vi "Write Single Coil.vi"(8 "error in":errorcluster, 9 "coil value":bool, 10 "address":u16, 11 "device data model in":refnum<class "Standard Data Model.lvclass">) -> (0 "error out":errorcluster, 3 "device data model out":refnum<class "Standard Data Model.lvclass">)   [LabVIEW 2021, in "Standard Data Model.lvclass"]
doc: "Writes the value of a single coil."
uses:
  Standard Data Model.lvclass
  Standard Data Model.lvclass/Standard Data Model.ctl
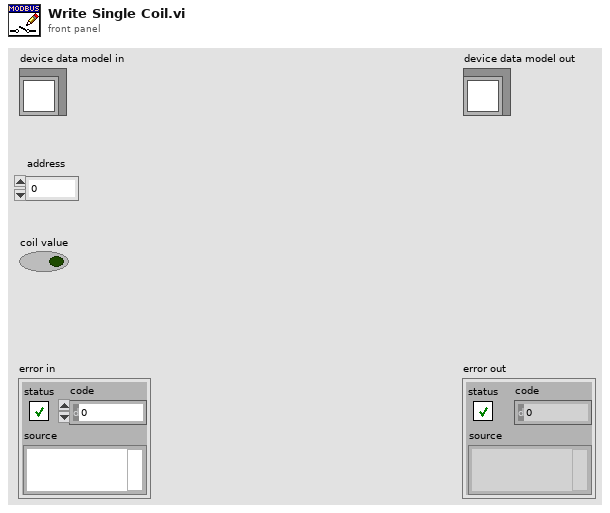
[diagram p1: front panel]
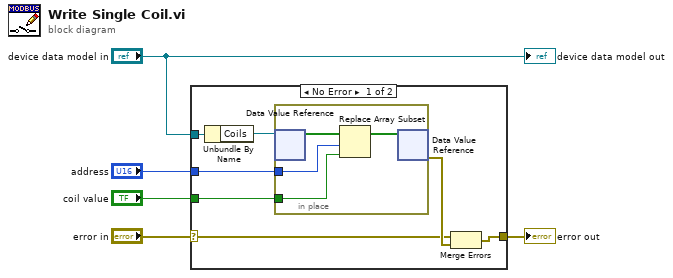
[diagram p0: block diagram]
diagram:
  n1 = case shown="No Error" "error in" {
    selector: "error in" -> [w6 w17]
    tunnel: "device data model in" -> [w12 _]
    tunnel: "coil value" -> [w10 _]
    tunnel: [w8 w17] -> w3
    tunnel: "address" -> [w7 _]
    frame No Error {
      n2 = Unbundle By Name(w12) -> ("Coils"=w11:refnum<data-value>)
      n3 = in-place {
        in-place-border: w10 -> [w14]
        in-place-border: w7 -> [w13]
        n4 = in-place-dvr #1(w11) -> (w16:bool[])  [unwired: 1 out]
        n5 = Replace Array Subset(array=w16, new element=w14, index=w13) -> (w15:bool[])
        n6 = in-place-dvr #1(w15) -> (w9:errorcluster)  [unwired: 1 out]
      }
      n7 = Merge Errors(w6, w9) -> (w8:errorcluster)
    }
    frame Error {
    }
  }
  "error out" <- w3
  "device data model out" <- "device data model in"
